vi "Cache.TestSteps.Write.vi"(7 "Idx":i32, 8 "error in (no error)":errorcluster, 10 "TS in":T1 {"TS"."TP"."value" format="%#.3f"; "TS"."TV"."minimum" format="%#.3f"; "TS"."TV"."maximum" format="%#.3f"}) -> (0 "error out":errorcluster)   [LabVIEW 2016]
uses:
  Cache.TestSteps.Fglb.TestData.ctl
  Database/ProdaNG/Controls/ProdaNG.Process.ctl
  Database/ProdaNG/Controls/ProdaNG.ProcessStep.ctl
  Database/ProdaNG/Controls/ProdaNG.ProcessStepParam.ctl
  Database/ProdaNG/Controls/ProdaNG.TestStep.ctl
  Database/ProdaNG/Controls/ProdaNG.TestValue.ctl
  Database/ProdaNG/Controls/ProdaNG.TestStepParam.ctl
  Database/ProdaNG/Controls/ProdaNG.Unit.ctl
  Global/ApplicationGlobal.vi
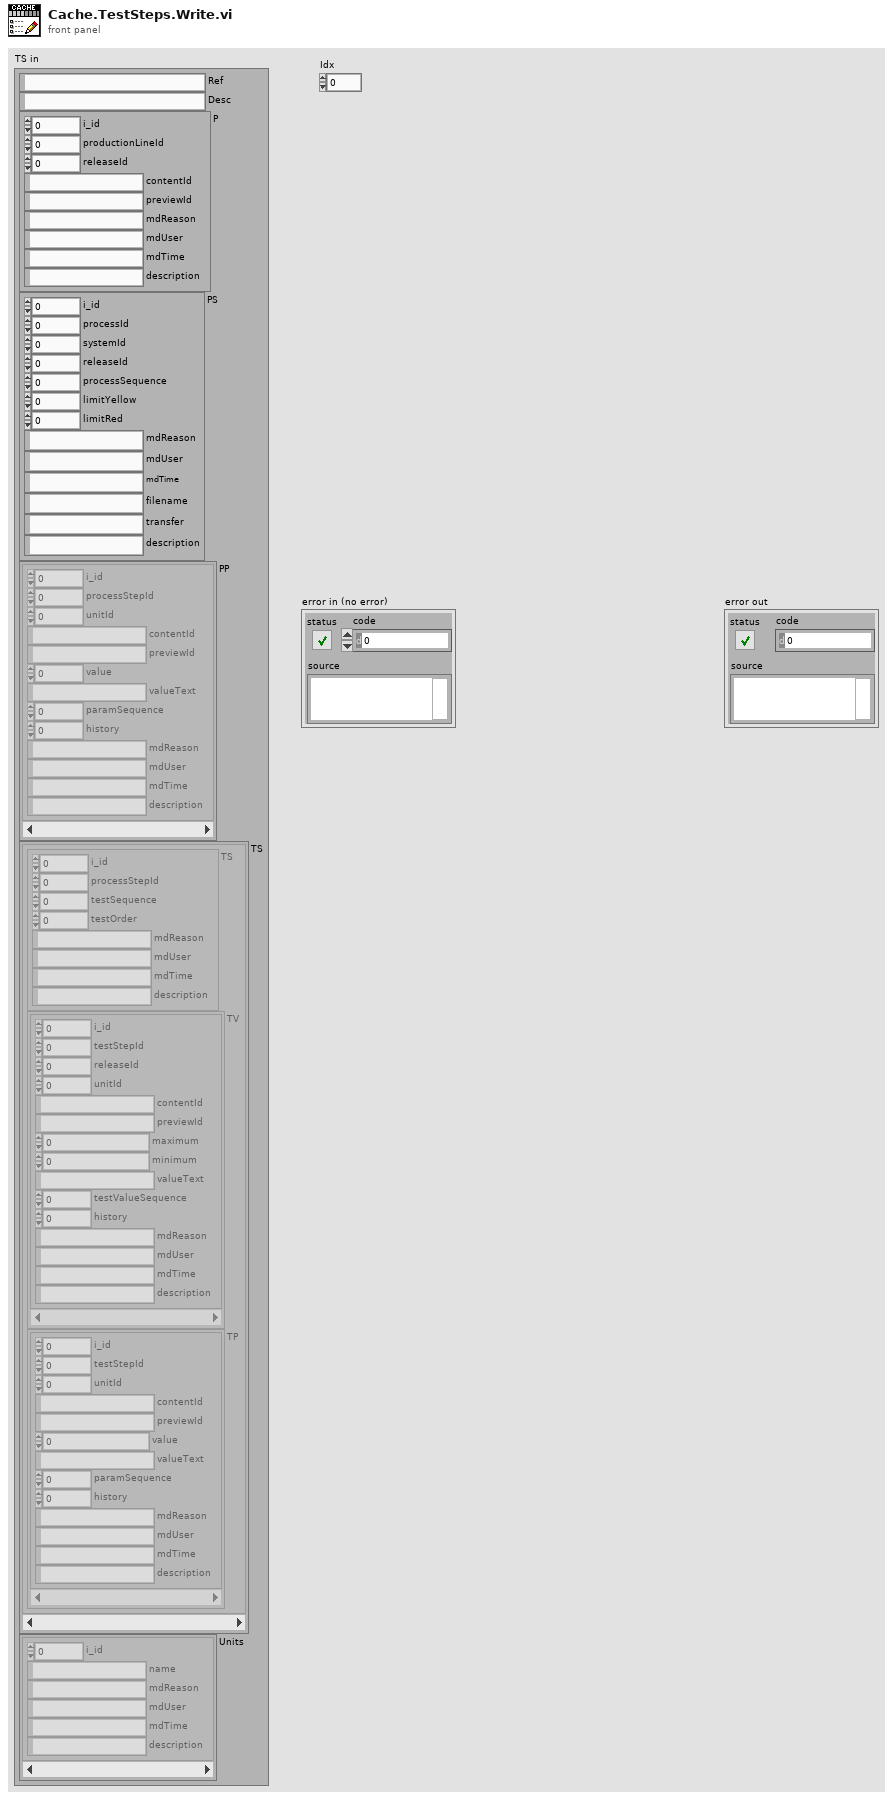
[diagram p1: front panel]
types:
  T1 = typedef "Cache.TestSteps.Fglb.TestData.ctl" = cluster{"Ref":string, "Desc":string, "P":T2, "PS":T3, "PP":T4[], "TS":cluster{"TS":T5, "TV":T6[], "TP":T7[]}[], "Units":T8[]}
  T2 = typedef "ProdaNG.Process.ctl" = cluster{"i_id":i32, "productionLineId":i32, "releaseId":i32, "contentId":string, "previewId":string, "mdReason":string, "mdUser":string, "mdTime":string, "description":string}
  T3 = typedef "ProdaNG.ProcessStep.ctl" = cluster{"i_id":i32, "processId":i32, "systemId":i32, "releaseId":i32, "processSequence":i32, "limitYellow":dbl, "limitRed":dbl, "mdReason":string, "mdUser":string, "mdTime":string, "filename":string, "transfer":string, "description":string}
  T4 = typedef "ProdaNG.ProcessStepParam.ctl" = cluster{"i_id":i32, "processStepId":i32, "unitId":i32, "contentId":string, "previewId":string, "value":dbl, "valueText":string, "paramSequence":i32, "history":i32, "mdReason":string, "mdUser":string, "mdTime":string, "description":string}
  T5 = typedef "ProdaNG.TestStep.ctl" = cluster{"i_id":i32, "processStepId":i32, "testSequence":i32, "testOrder":i32, "mdReason":string, "mdUser":string, "mdTime":string, "description":string}
  T6 = typedef "ProdaNG.TestValue.ctl" = cluster{"i_id":i32, "testStepId":i32, "releaseId":i32, "unitId":i32, "contentId":string, "previewId":string, "maximum":dbl, "minimum":dbl, "valueText":string, "testValueSequence":i32, "history":i32, "mdReason":string, "mdUser":string, "mdTime":string, "description":string}
  T7 = typedef "ProdaNG.TestStepParam.ctl" = cluster{"i_id":i32, "testStepId":i32, "unitId":i32, "contentId":string, "previewId":string, "value":dbl, "valueText":string, "paramSequence":i32, "history":i32, "mdReason":string, "mdUser":string, "mdTime":string, "description":string}
  T8 = typedef "ProdaNG.Unit.ctl" = cluster{"i_id":i32, "name":string, "mdReason":string, "mdUser":string, "mdTime":string, "description":string}
  T9 = enum16{"open", "replace", "create", "open or create", "replace or create", "replace or create with confirmation"}
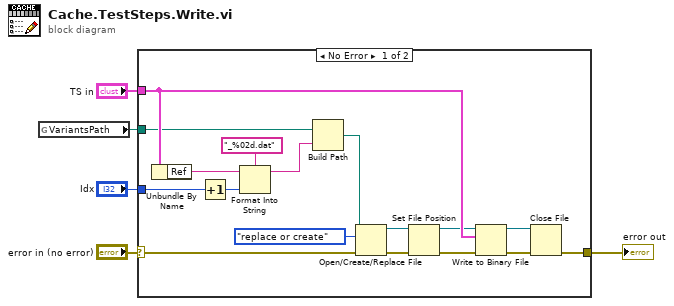
[diagram p0: block diagram]
diagram:
  n1 = global read "ApplicationGlobal.vi" "VariantsPath"() -> (w2:path)
  n2 = case shown="No Error" "error in (no error)" {
    selector: "error in (no error)" -> [w9 w23]
    tunnel: "TS in" -> [w22 _]
    tunnel: [w21 w23] -> w5
    tunnel: "Idx" -> [w14 _]
    tunnel: w2 -> [w8 _]
    frame No Error {
      n3 = Unbundle By Name(w22) -> ("Ref"=w11:string)
      n4 = Increment(x=w14) -> (x+1=w6:i32)
      n5 = Format Into String(format string="_%02d.dat", initial string=w11, w6) -> (resulting string=w7:string)  [unwired: 1 in, 1 out]
      n6 = Build Path(base path=w8, name or relative path=w7) -> (appended path=w13:path)
      n7 = Open/Create/Replace File(file path (use dialog)=w13, error in=w9, operation (0:open)=T9."replace or create") -> (refnum out=w19:refnum<file>, error out=w17:errorcluster)  [unwired: 3 in, 1 out]
      n8 = Set File Position(refnum=w19, error in=w17) -> (refnum out=w18:refnum<file>, error out=w16:errorcluster)  [unwired: 2 in]
      n9 = Write to Binary File(file (use dialog)=w18, data=w22, error in=w16) -> (refnum out=w20:refnum<file>, error out=w15:errorcluster)  [unwired: 3 in, 1 out]
      n10 = Close File(refnum=w20, error in=w15) -> (error out=w21:errorcluster)  [unwired: 1 out]
    }
    frame Error {
    }
  }
  "error out" <- w5
